vi "N-View.vi"(8 "error in":errorcluster, 11 "Q Name":string) -> (0 "error out":errorcluster, 2 "Waveform":waveform(dbl)[](array[waveform]))   [LabVIEW 2016]
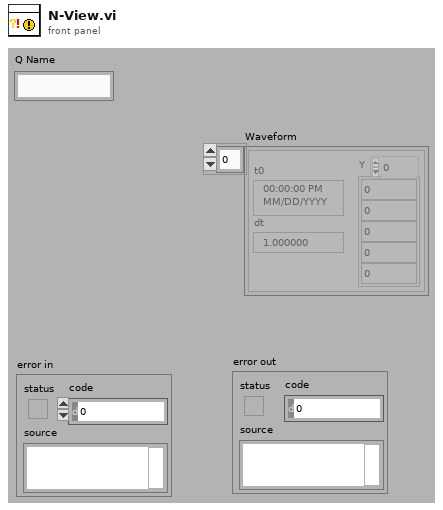
[diagram p1: front panel]
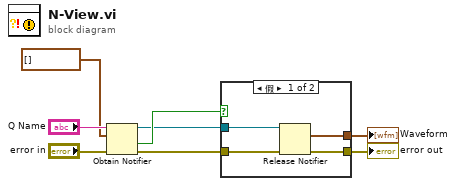
[diagram p0: block diagram]
diagram:
  n1 = Obtain Notifier(name (unnamed)="Q Name", notification data type=waveform(dbl)[] [] ("Waveform"), error in (no error)="error in") -> (notifier out=w2:refnum<notifier>, created new?=w6:bool, error out=w3:errorcluster)  [unwired: 1 in]
  n2 = case shown="假" w6 {
    tunnel: w2 -> [w12 _]
    tunnel: w3 -> [w11 w13]
    tunnel: [w10 w13] -> w5
    tunnel: [w9 _] -> w1
    frame False {
      n3 = Release Notifier(notifier=w12, error in (no error)=w11) -> (last notification=w9:waveform(dbl)[], error out=w10:errorcluster)  [unwired: 1 in, 1 out]
    }
    frame True {
    }
  }
  "error out" <- w5
  "Waveform" <- w1
